vi "Load Waveform From TDMS.vi"(0 "TDMS File Path":path, 5 "Waveform Name (File Name)":string, 11 "error in (no error)":errorcluster) -> (4 "Waveform":T1={"Name"="Wfm", "Data"=refnum, "Signal Bandwidth (Hz)"=0.0, "PAPR (dB)"=0.0, "Burst Length (s)"=0.0, "Sample Rate"=0.0, "Burst Start Locations"=[], "Burst Stop Locations"=[], "Idle Duration Present?"=FALSE, "Runtime Scaling"=0.0, "Script"=""} {"Runtime Scaling" format="%#_6p"; "Sample Rate" format="%#_6p"; "Burst Length (s)" format="%#_6p"; "PAPR (dB)" format="%.2f"; "Signal Bandwidth (Hz)" format="%.2f"}, 15 "error out":errorcluster)   [LabVIEW 2019, in "SG.lvlib"]
doc: "Loads a waveform and relevant properties from a TDMS file."
uses:
  SG.lvlib
  Common/Waveform.ctl
  <instrlib>/niRFSGPlayback/niRFSGPlayback Read Waveform From File (1 Wfm,TDMS, CSG).vi
  Common/Common.lvlib
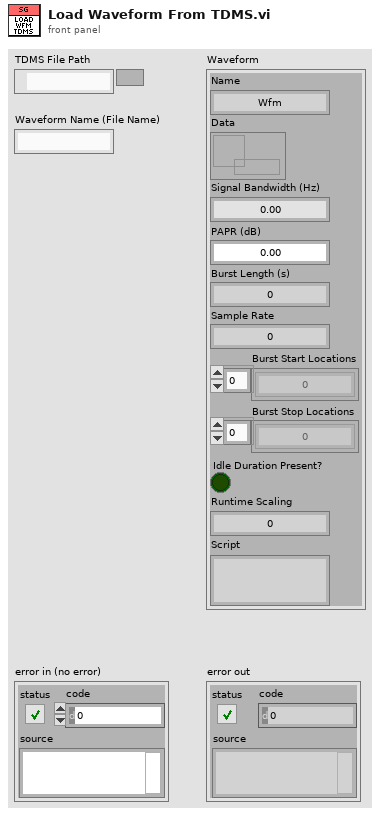
[diagram p1: front panel]
types:
  T1 = typedef "Common.lvlib/Waveform.ctl" = cluster{"Name":string, "Data":refnum<data-value>, "Signal Bandwidth (Hz)":dbl, "PAPR (dB)":dbl, "Burst Length (s)":dbl, "Sample Rate":dbl, "Burst Start Locations":i32[], "Burst Stop Locations":i32[], "Idle Duration Present?":bool, "Runtime Scaling":dbl, "Script":string}
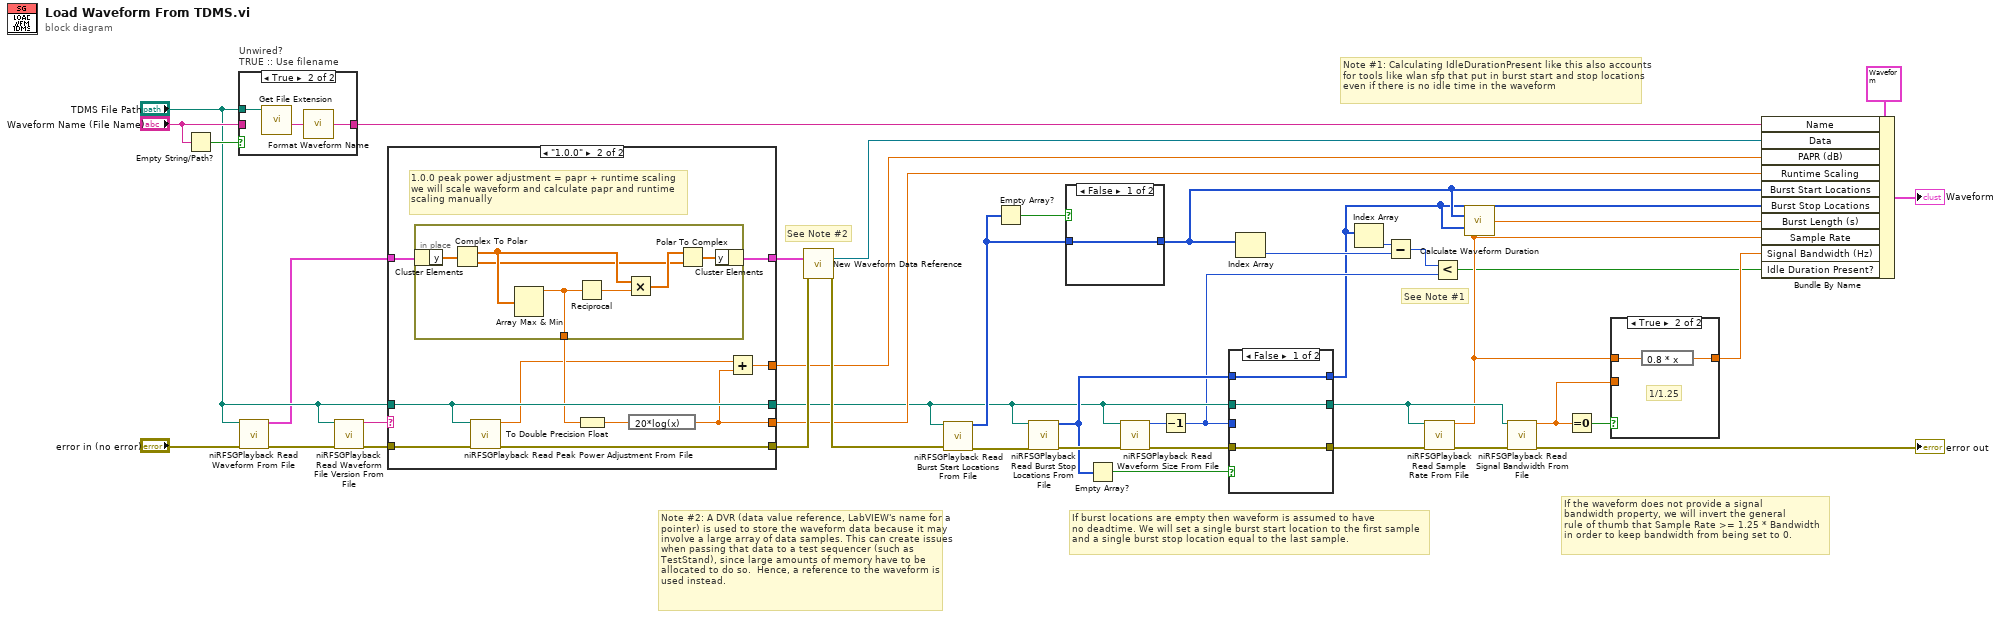
[diagram p0: block diagram]
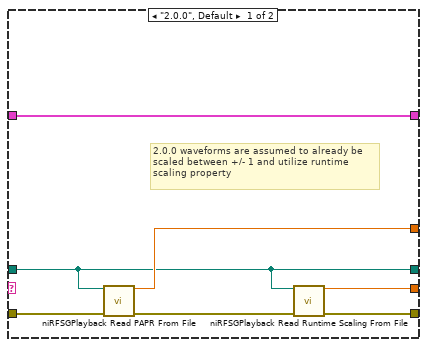
[diagram p2: hidden frame]
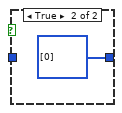
[diagram p4: hidden frame]
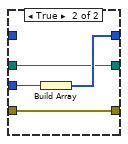
[diagram p5: hidden frame]
diagram:
  # "See Note #2"
  # "Note #2: A DVR (data value reference, LabVIEW's name for a pointer) is used to store the waveform data because it may involve a large array of data samples. This can create issues when passing that data to a test sequencer (such as TestStand), since large amounts of memory have to be allocated to do so.  Hence, a reference to the waveform is used instead."
  # "See Note #1"
  # "Note #1: Calculating IdleDurationPresent like this also accounts for tools like wlan sfp that put in burst start and stop locations even if there is no idle time in the waveform"
  # "If the waveform does not provide a signal\nbandwidth property, we will invert the general\nrule of thumb that Sample Rate >= 1.25 * Bandwidth\nin order to keep bandwidth from being set to 0."
  # "If burst locations are empty then waveform is assumed to have\nno deadtime. We will set a single burst start location to the first sample \nand a single burst stop location equal to the last sample."
  n1 = Empty String/Path?(string/path="Waveform Name (File Name)") -> (empty?=w29:bool)
  n2 = case "Unwired?\nTRUE :: Use filename" shown="True" w29 {
    tunnel: [w43 w44] -> w27
    tunnel: "Waveform Name (File Name)" -> [w43 _]
    tunnel: "TDMS File Path" -> [_ w46]
    frame False {
    }
    frame True {
      n3 = call <vilib>:"Get File Extension.vi"("file"=w46) -> ("filename without extension"=w45:string)  [unwired: 6 in, 4 out]
      n4 = call "Format Waveform Name.vi"("Waveform File Name"=w45) -> ("Waveform Name"=w44:string)
    }
  }
  n5 = call-poly <instrlib>:"niRFSGPlayback Read Waveform From File.vi"("file path"="TDMS File Path", "error in"="error in (no error)") -> ("waveform"=w18:cluster{"t0":dbl, "dt":dbl, "y":csg[]}, "error out"=w41:errorcluster)  [unwired: 12 in]
  n6 = call <instrlib>:"niRFSGPlayback Read Waveform File Version From File.vi"("file path"="TDMS File Path", "error in"=w41) -> ("waveform file version"=w31:string, "error out"=w40:errorcluster)  [unwired: 12 in]
  n7 = case shown="\"1.0.0\"" w31 {
    tunnel: w40 -> [w53 w63]
    tunnel: [w49 w61] -> w8
    tunnel: [w50 w54] -> w30
    tunnel: "TDMS File Path" -> [w49 w61]
    tunnel: [w48 w55] -> w19
    tunnel: w18 -> [w47 w60]
    tunnel: [w47 w59] -> w1
    tunnel: [w51 w62] -> w33
    frame "2.0.0", Default {
      # "2.0.0 waveforms are assumed to already be\nscaled between +/- 1 and utilize runtime\nscaling property"
      n8 = call <instrlib>:"niRFSGPlayback Read PAPR From File.vi"("file path"=w49, "error in"=w53) -> ("PAPR"=w50:dbl, "error out"=w52:errorcluster)  [unwired: 12 in]
      n9 = call <instrlib>:"niRFSGPlayback Read Runtime Scaling From File.vi"("file path"=w49, "error in"=w52) -> ("runtime scaling"=w48:dbl, "error out"=w51:errorcluster)  [unwired: 12 in]
    }
    frame "1.0.0" {
      # "1.0.0 peak power adjustment = papr + runtime scaling\nwe will scale waveform and calculate papr and runtime\nscaling manually"
      n10 = in-place {
        in-place-border: [w66] -> w58
        n11 = in-place-cluster #1(w60) -> ("y"=w65:csg[])
        n12 = Complex To Polar(r * e^(i*theta)=w65) -> (r=w69:sgl[], theta=w68:sgl[])
        n13 = Array Max & Min(array=w69) -> (max value=w66:sgl)  [unwired: 3 out]
        n14 = Reciprocal(x=w66) -> (1/x=w64:sgl)
        n15 = Multiply(x=w69, y=w64) -> (x*y=w70:sgl[])
        n16 = Polar To Complex(1:w68, 2:w70) -> (0:w67:csg[])
        n17 = in-place-cluster #1("y"=w67) -> (w59:cluster{"t0":dbl, "dt":dbl, "y":csg[]})
      }
      n18 = call <instrlib>:"niRFSGPlayback Read Peak Power Adjustment From File.vi"("file path"=w61, "error in"=w63) -> ("peak power adjustment"=w56:dbl, "error out"=w62:errorcluster)  [unwired: 12 in]
      n19 = To Double Precision Float(number=w58) -> (double precision float=w57:dbl)
      n20 = expression code="20*log(x)"(w57) -> (w55:dbl)
      n21 = Add(x=w56, y=w55) -> (x+y=w54:dbl)
    }
  }
  n22 = call "New Waveform Data Reference.vi"("Waveform Data"=w1, "error in (no error)"=w33) -> ("Waveform Data Reference"=w2:refnum<data-value>, "error out"=w32:errorcluster)  [unwired: 12 in]
  n23 = call <instrlib>:"niRFSGPlayback Read Burst Start Locations From File.vi"("file path"=w8, "error in"=w32) -> ("burst start locations"=w23:i32[], "error out"=w39:errorcluster)  [unwired: 12 in]
  n24 = Empty Array?(array=w23) -> (empty?=w24:bool)
  n25 = call <instrlib>:"niRFSGPlayback Read Burst Stop Locations From File.vi"("file path"=w8, "error in"=w39) -> ("burst stop locations"=w21:i32[], "error out"=w35:errorcluster)  [unwired: 12 in]
  n26 = case shown="False" w24 {
    tunnel: w23 -> [w71 _]
    tunnel: [w71 i32[] [0]] -> w11
    frame False {
    }
    frame True {
    }
  }
  n27 = Empty Array?(array=w21) -> (empty?=w22:bool)
  n28 = call <instrlib>:"niRFSGPlayback Read Waveform Size From File.vi"("file path"=w8, "error in"=w35) -> ("waveform size"=w7:i32, "error out"=w34:errorcluster)  [unwired: 12 in]
  n29 = Decrement(x=w7) -> (x-1=w6:i32)
  n30 = case shown="False" w22 {
    tunnel: w8 -> [w73 w77]
    tunnel: w34 -> [w75 w79]
    tunnel: [w75 w79] -> w37
    tunnel: w21 -> [w74 _]
    tunnel: [w74 w78] -> w4
    tunnel: [w73 w77] -> w20
    tunnel: w6 -> [_ w76]
    frame False {
    }
    frame True {
      n31 = Build Array(w76) -> (w78:i32[])
    }
  }
  n32 = Index Array(array=w11) -> (element=w10:i32)  [unwired: 1 in]
  n33 = Index Array(array=w4) -> (element=w9:i32)  [unwired: 1 in]
  n34 = Subtract(x=w9, y=w10) -> (x-y=w3:i32)
  n35 = call <instrlib>:"niRFSGPlayback Read Sample Rate From File.vi"("file path"=w20, "error in"=w37) -> ("sample rate"=w12:dbl, "error out"=w38:errorcluster)  [unwired: 12 in]
  n36 = Less?(x=w3, y=w6) -> (x < y?=w5:bool)
  n37 = call "Calculate Waveform Duration.vi"("Sample Rate"=w12, "Burst Start Locations"=w11, "Burst Stop Locations"=w4) -> ("Burst Length (s)"=w13:dbl)  [unwired: 12 in]
  n38 = call <instrlib>:"niRFSGPlayback Read Signal Bandwidth From File.vi"("file path"=w20, "error in"=w38) -> ("signal bandwidth"=w15:dbl, "error out"=→"error out":errorcluster)  [unwired: 12 in]
  n39 = Equal To 0?(x=w15) -> (x = 0?=w16:bool)
  n40 = case shown="True" w16 {
    tunnel: w12 -> [_ w82]
    tunnel: w15 -> [w80 _]
    tunnel: [w80 w81] -> w14
    frame False {
    }
    frame True {
      # "1/1.25"
      n41 = expression code="0.8 * x"(w82) -> (w81:dbl)
    }
  }
  n42 = Bundle By Name(cluster=T1 {"Name"="Wfm", "Data"=refnum, "Signal Bandwidth (Hz)"=0.0, "PAPR (dB)"=0.0, "Burst Length (s)"=0.0, "Sample Rate"=0.0, "Burst Start Locations"=[], "Burst Stop Locations"=[], "Idle Duration Present?"=FALSE, "Runtime Scaling"=0.0, "Script"=""} ("Waveform"), "Name"=w27, "Data"=w2, "PAPR (dB)"=w30, "Runtime Scaling"=w19, "Burst Start Locations"=w11, "Burst Stop Locations"=w4, "Burst Length (s)"=w13, "Sample Rate"=w12, "Signal Bandwidth (Hz)"=w14, "Idle Duration Present?"=w5) -> (→"Waveform":T1)
